vi "ㄴㄷㅎㄶ.vi"() -> ()   [LabVIEW 2015]
uses:
  <vilib>/NXT/Block Support/NXT_InputPort.ctl
  <vilib>/NXT/Subs/MotorOutput.ctl
  <vilib>/NXT/Dual Mode Library/Sensors/Light_On.vi
  <vilib>/NXT/Dual Mode Library/Motors/MotorOn.vi
  <vilib>/NXT/Dual Mode Library/Waits/Wait_Num.vi
  <vilib>/NXT/Dual Mode Library/Motors/MotorReverse.vi
  <vilib>/NXT/Dual Mode Library/Motors/Rotation.vi
panel:
  in  "Time (1 sec) 2":sgl=1.0
  in  "Time (1 sec)":sgl=1.0
  in  "Angle of Rotation":i32
  in  "Power (75)":i32=75
  in  "stop":bool
  in  "Power/Speed 1":i8=75
  in  "왼쪽빛":T1=2 items=["Port 1", "Port 2", "Port 3", "Port 4"]
  in  "오른쪽 빛":T1=2 items=["Port 1", "Port 2", "Port 3", "Port 4"]
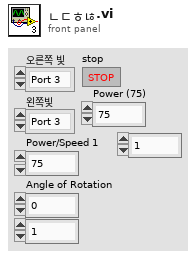
[diagram p1: front panel]
types:
  T1 = typedef "NXT_InputPort.ctl" = u32
  T2 = typedef "MotorOutput.ctl" = u8
  T3 = typedef "LVHSConnector.ctl" = refnum<class "BrickReference.lvclass">
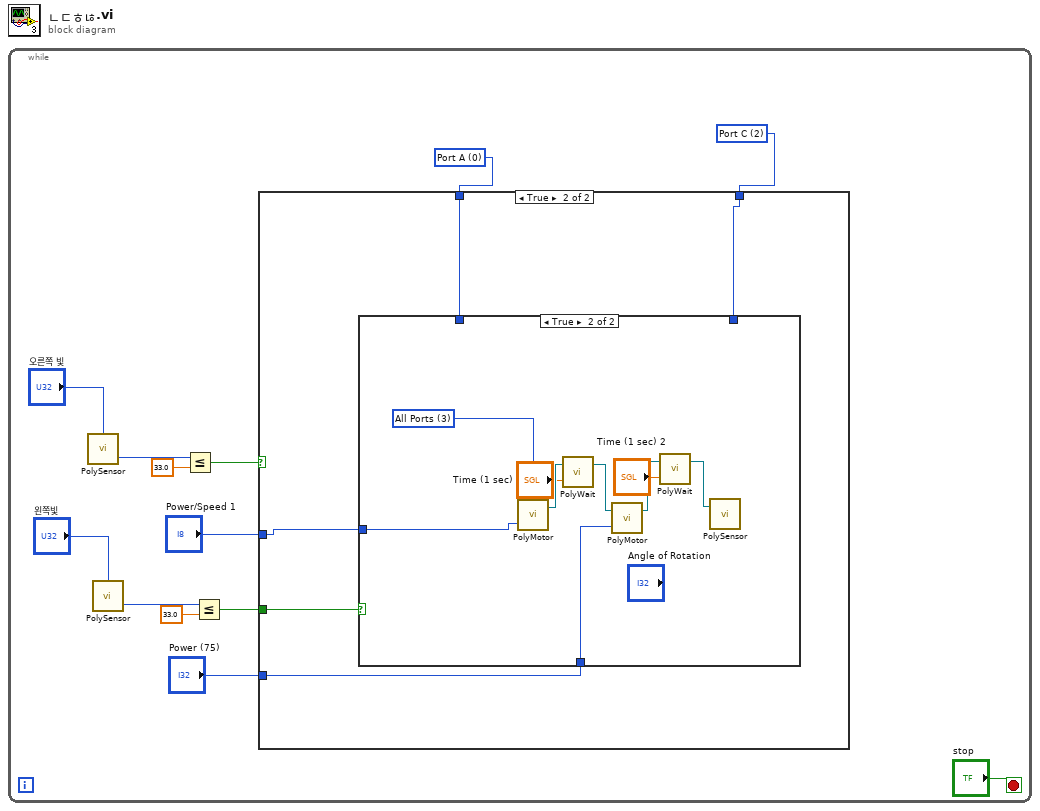
[diagram p0: block diagram]
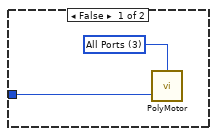
[diagram p3: hidden frame]
diagram:
  n1 = while {
    stop <- "stop" stop-if-true
    w3 = T2 0 items=["Port A"=0, "Port B"=1, "Port C"=2, "Ports A & B"=4, "Ports A & C"=5, "Ports B & C"=6, "All Ports"=3] ("Output Port (All Ports)")
    w2 = T2 2 items=["Port A"=0, "Port B"=1, "Port C"=2, "Ports A & B"=4, "Ports A & C"=5, "Ports B & C"=6, "All Ports"=3] ("Output Port (All Ports)")
    n2 = call-poly <vilib>:"PolySensor.vi"("Port (Port 3)"="오른쪽 빛") -> ("Scaled Value"=w8:i16)  [unwired: 2 in, 1 out]
    n3 = call-poly <vilib>:"PolySensor.vi"("Port (Port 3)"="왼쪽빛") -> ("Scaled Value"=w7:i16)  [unwired: 2 in, 1 out]
    n4 = Less Or Equal?(x=w8, y=33.0) -> (x <= y?=w11:bool)
    n5 = Less Or Equal?(x=w7, y=33.0) -> (x <= y?=w6:bool)
    n6 = case shown="True" w11 {
      tunnel: w6 -> [_ w17]
      tunnel: "Power/Speed 1" -> [_ w18]
      tunnel: w2 -> [_ w16]
      tunnel: w3 -> [_ w15]
      tunnel: "Power (75)" -> [_ w14]
      frame False {
      }
      frame True {
        n7 = case shown="True" w17 {
          tunnel: w18 -> [w20 w29]
          tunnel: w16 -> [_ _]
          tunnel: w15 -> [_ _]
          tunnel: w14 -> [_ w23]
          frame False {
            w19 = T2 3 items=["Port A"=0, "Port B"=1, "Port C"=2, "Ports A & B"=4, "Ports A & C"=5, "Ports B & C"=6, "All Ports"=3] ("Output Port (All Ports)")
            n8 = call-poly <vilib>:"PolyMotor.vi"("Power (75)"=w20, "Output Port (All Ports)"=w19) -> ()  [unwired: 1 in, 2 out]
          }
          frame True {
            w28 = T2 3 items=["Port A"=0, "Port B"=1, "Port C"=2, "Ports A & B"=4, "Ports A & C"=5, "Ports B & C"=6, "All Ports"=3] ("Output Port (All Ports)")
            n9 = call-poly <vilib>:"PolyMotor.vi"("Power (75)"=w29, "Output Port (All Ports)"=w28) -> ("NXT/EV3"=w27:T3)  [unwired: 1 in, 1 out]
            n10 = call-poly <vilib>:"PolyWait.vi"("Time (1 sec)"="Time (1 sec)", "NXT/EV3"=w27) -> ("NXT/EV3"=w26:T3)  [unwired: 2 in]
            n11 = call-poly <vilib>:"PolyMotor.vi"("Power (75)"=w23, "NXT/EV3"=w26) -> ("NXT/EV3"=w25:T3)  [unwired: 1 in, 1 out]
            n12 = call-poly <vilib>:"PolyWait.vi"("Time (1 sec)"="Time (1 sec) 2", "NXT/EV3"=w25) -> ("NXT/EV3"=w24:T3)  [unwired: 2 in]
            n13 = call-poly <vilib>:"PolySensor.vi"("NXT/EV3"=w24) -> ()  [unwired: 1 in, 3 out]
          }
        }
      }
    }
  }
